vi "Post-Build Action.vi"(5 "Files Generated by Build":path[](array[path]), 6 "Top Level/Always Included VIs":path[](array[path]), 7 "Destination Path":path, 8 "error in (no error)":errorcluster, 9 "Target Name":string, 10 "Build Specification Name":string, 11 "Project Path":path) -> (0 "error out":errorcluster)   [LabVIEW 2015]
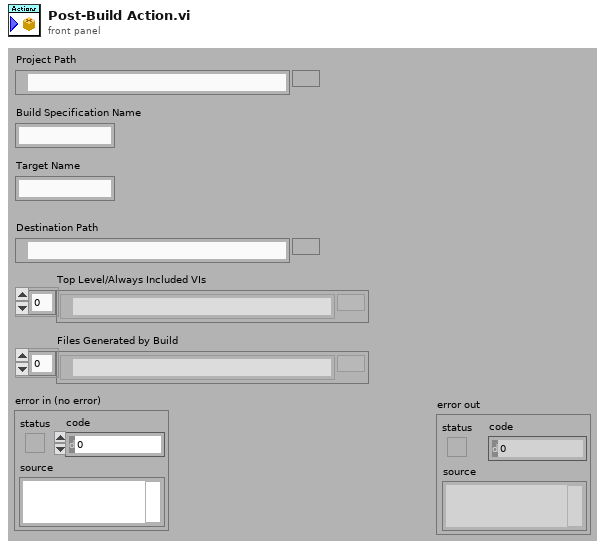
[diagram p1: front panel]
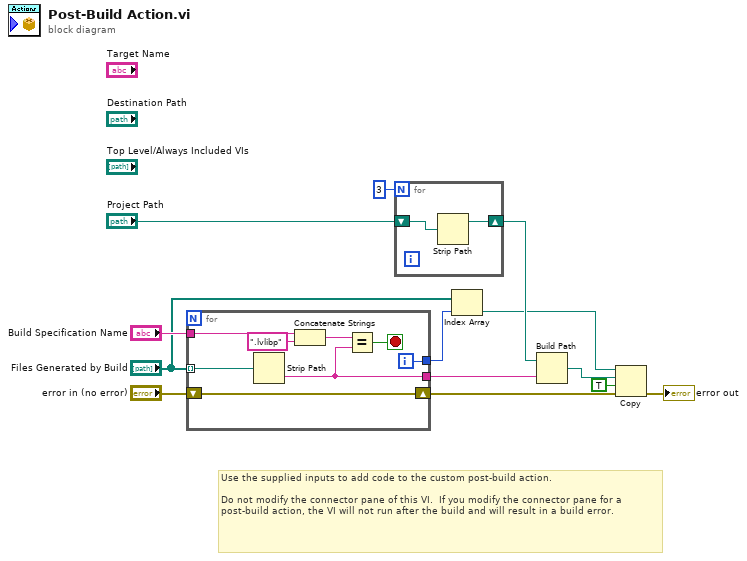
[diagram p0: block diagram]
diagram:
  # "Use the supplied inputs to add code to the custom post-build action.\n\nDo not modify the connector pane of this VI.  If you modify the connector pane for a post-build action, the VI will not run after the build and will result in a build error."
  n1 = for {
    tunnel: "Files Generated by Build" -> [w18] mode=indexing
    shift-right: [w19] -> w5
    shift-left: "error in (no error)" -> [w19]
    tunnel: "Build Specification Name" -> [w17]
    tunnel: [w20] -> w10
    tunnel: [w14] -> w6
    i -> [w20]
    stop <- w21 stop-if-true
    n2 = Strip Path(path=w18) -> (name=w14:string)  [unwired: 1 out]
    n3 = Concatenate Strings(w17, ".lvlibp" ("string")) -> (w16:string)
    n4 = Equal?(x=w16, y=w14) -> (x = y?=w21:bool)
  }
  n5 = for {
    N: 3 -> [_]
    shift-right: [w22] -> w7
    shift-left: "Project Path" -> [w23]
    n6 = Strip Path(path=w23) -> (stripped path=w22:path)  [unwired: 1 out]
  }
  n7 = Index Array(array="Files Generated by Build", index=w10) -> (element=w3:path)
  n8 = Build Path(base path=w7, name or relative path=w6) -> (appended path=w2:path)
  n9 = Copy(8:w5, 9:TRUE ("overwrite (F)"), 10:w2, 11:w3) -> (0:→"error out":errorcluster)  [unwired: 1 in, 2 out]
